vi "PH_AxisGUI_6P.CheckInterface.vi"(0 "i ref in":refnum<vi>, 5 "error in":errorcluster) -> (14 "i ref out":refnum<vi>, 19 "error out":errorcluster)   [LabVIEW 2009]
uses:
  PH_AxisGUI_6P.lvlib
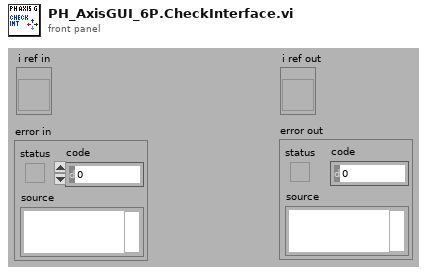
[diagram p1: front panel]
types:
  T1 = typedef "PH_AxisGUI_6P.lvlib/PH_AxisGUI_6P.i attribute.ctl" = cluster{"Axis1":T2, "Axis2":T2, "GUI Refs":cluster{"UP":refnum<vi>, "DOWN":refnum<vi>, "LEFT":refnum<vi>, "RIGHT":refnum<vi>, "Axis1_Status":refnum<vi>, "Axis2_Status":refnum<vi>, "Axis1_Target":refnum<vi>, "Axis2_Target":refnum<vi>, "Axis1_Position":refnum<vi>, "Axis2_Position":refnum<vi>, "Axis1_Information":refnum<vi>, "Axis2_Information":refnum<vi>, "Axis1_Advanced":refnum<vi>, "Axis2_Advanced":refnum<vi>, "AxisSelection":refnum<vi>, "Keys":refnum<vi>, "Tab Control":refnum<vi>, "StopMotor":refnum<vi>, "SetZero":refnum<vi>, "Reset Controller":refnum<vi>, "Axis1_Status Bar":refnum<vi>, "Axis2_Status Bar":refnum<vi>, "Axis1_Scale":refnum<vi>, "Axis2_Scale":refnum<vi>}, "Up-Label":string, "Down-Label":string, "Left-Label":string, "Right-Label":string, "GUI Manager Path":string}
  T2 = typedef "PH_AxisGUI_6P.lvlib/PH_AxisGUI_6P.AxisInformation.ctl" = cluster{"SixPack Instance":string, "Motor Nr":i32, "Axis Name":string, "Moving":bool, "State":T3}
  T3 = typedef "PH_AxisGUI_6P.lvlib/PH_AxisGUI_6P.AxisState.ctl" = enum16{"NoLink", "Inactive", "Active", "Error", "NoInfo"}
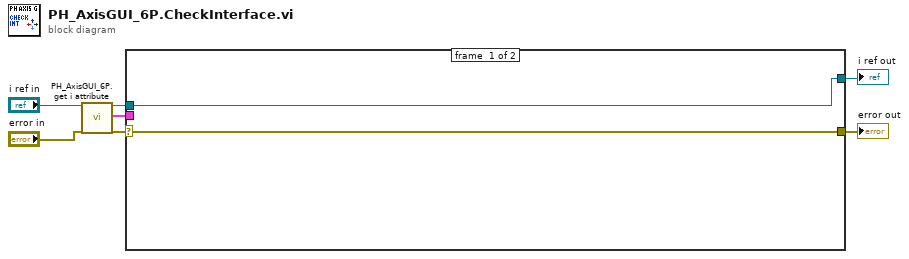
[diagram p0: block diagram]
diagram:
  n1 = call "PH_AxisGUI_6P.get i attribute.vi"("i ref in"="i ref in", "error in (no error)"="error in") -> ("i ref out"=w4:refnum<vi>, "i attribute"=w1:T1, "error out"=w2:errorcluster)  [unwired: 15 in]
  n2 = case shown="No Error" w2 {
    selector: w2 -> [w8 w11]
    tunnel: w4 -> [w9 w10]
    tunnel: [w9 w10] -> w7
    tunnel: [w8 w11] -> w6
    tunnel: w1 -> [_ _]
    frame #0 {
    }
    frame #1 {
    }
  }
  "error out" <- w6
  "i ref out" <- w7
